vi "Resideo Close.vi"(8 "error in (no error)":errorcluster, 11 "Modbus Master in":refnum<class "Modbus Master.lvclass">) -> (0 "error out":errorcluster)   [LabVIEW 2023]
uses:
  <vilib>/NI/Modbus Library/API/Master/Modbus Master.lvclass
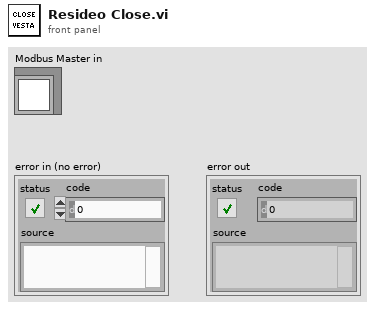
[diagram p1: front panel]
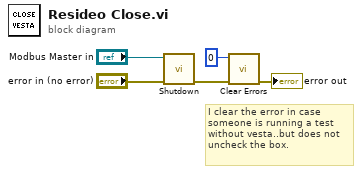
[diagram p0: block diagram]
diagram:
  # "I clear the error in case\nsomeone is running a test\nwithout vesta..but does not\nuncheck the box."
  n1 = call-dynamic "Shutdown.vi"("error in"="error in (no error)", "Modbus master in"="Modbus Master in") -> ("error out"=w2:errorcluster)  [unwired: 9 in]
  n2 = call <vilib>:"Clear Errors.vi"("error in (no error)"=w2, "specific error code to clear (0: all)"=0) -> ("error out"=→"error out":errorcluster)  [unwired: 4 in, 1 out]
